vi "Get Cache Path.vi"(8 "error in":errorcluster, 11 "Path Getter in":refnum<class "Path Getter.lvclass">) -> (0 "error out":errorcluster, 2 "Path":path)   [LabVIEW 2020, in "Path Getter.lvclass"]
doc: "Retrieves path of <b>Cache File</b>."
uses:
  Path Getter.lvclass
  Path Getter.lvclass/Path Getter.ctl
  <resource>/dialog/lvconfig.llb/LV Config Read String.vi
  <resource>/dialog/lvconfig.llb/LV Config Write String.vi
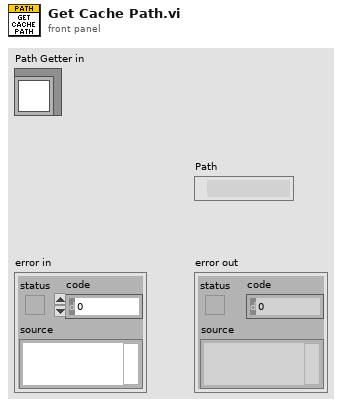
[diagram p1: front panel]
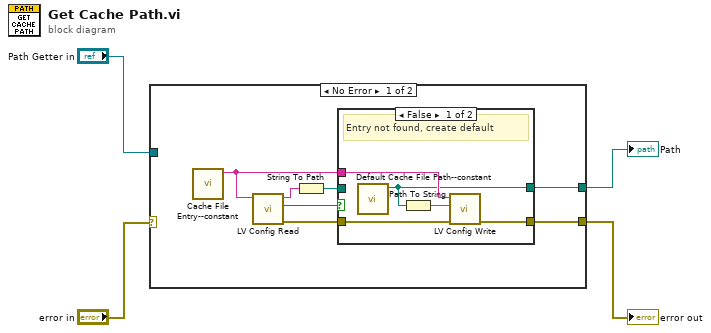
[diagram p0: block diagram]
diagram:
  n1 = case shown="No Error" "error in" {
    selector: "error in" -> [_ w19]
    tunnel: [w10 w19] -> w4
    tunnel: [w5 _] -> w2
    tunnel: "Path Getter in" -> [_ _]
    frame No Error {
      n2 = call "Cache File Entry--constant.vi"() -> ("Entry"=w7:string)  [unwired: 11 in]
      n3 = call-poly <resource>:"LV Config Read.vi"("key"=w7) -> ("error out"=w11:errorcluster, "found?"=w6:bool, "value"=w8:string)  [unwired: 4 in]
      n4 = String To Path(string=w8) -> (path=w9:path)
      n5 = case shown="False" w6 {
        tunnel: w7 -> [w14 _]
        tunnel: w11 -> [w16 w18]
        tunnel: w9 -> [_ w17]
        tunnel: [w12 w17] -> w5
        tunnel: [w15 w18] -> w10
        frame False {
          # "Entry not found, create default"
          n6 = call "Default Cache File Path--constant.vi"() -> ("appended path"=w12:path)  [unwired: 11 in]
          n7 = Path To String(path=w12) -> (string=w13:string)
          n8 = call-poly <resource>:"LV Config Write.vi"("error in (no error)"=w16, "value"=w13, "key"=w14) -> ("error out"=w15:errorcluster)  [unwired: 4 in]
        }
        frame True {
          # "Entry found --> Use value"
        }
      }
    }
    frame Error {
      # "Pass error without further action"
    }
  }
  "error out" <- w4
  "Path" <- w2
